vi "6009_short.vi"() -> ()   [LabVIEW 2009]
panel:
  out "Waveform Graph 2":dynamicdata(graph)
  out "Waveform Graph":dynamicdata(graph)
  in  "stop (F)":bool
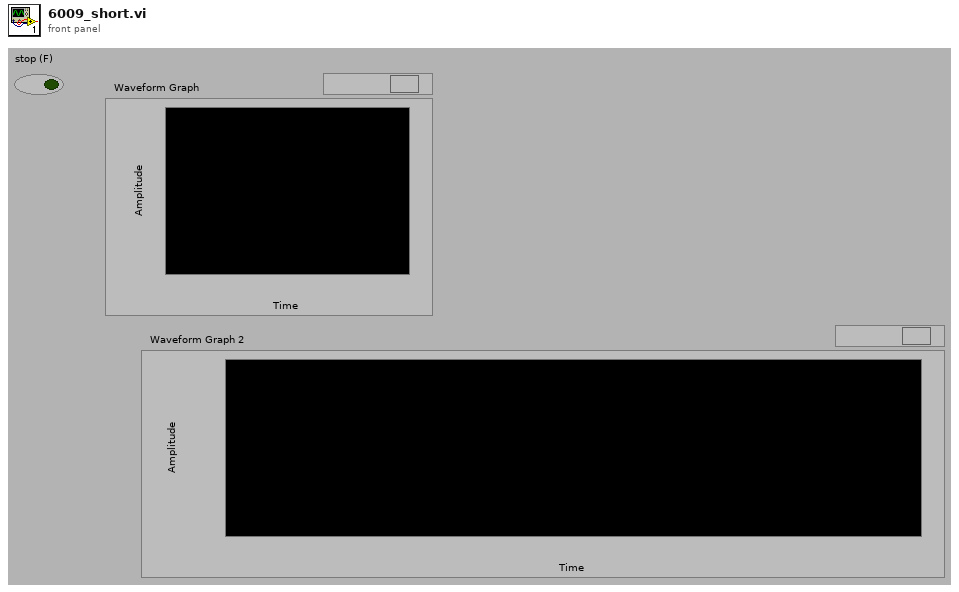
[diagram p1: front panel]
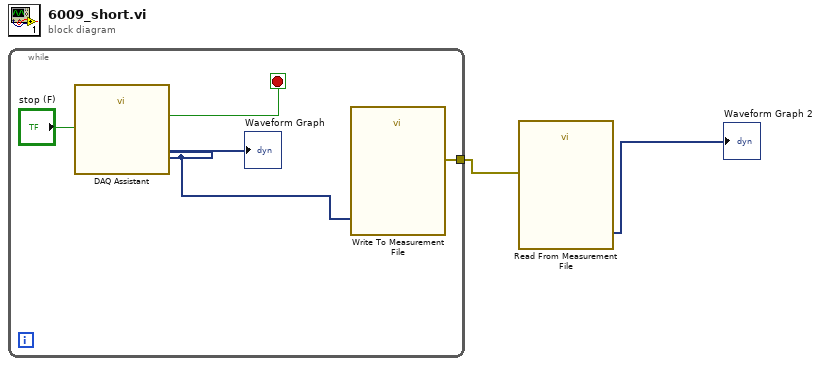
[diagram p0: block diagram]
diagram:
  n1 = while {
    tunnel: [w3] -> w2
    stop <- w5 stop-if-true
    n2 = call "DAQ Assistant"("stop (F)"="stop (F)") -> ("data"=w4:dynamicdata, "stopped"=w5:bool)  [unwired: 15 in, 2 out]
    "Waveform Graph" <- w4
    n3 = call "Write To Measurement File"("Signals"=w4) -> ("error out"=w3:errorcluster)  [unwired: 16 in, 2 out]
  }
  n4 = call "Read From Measurement File"("error in (no error)"=w2) -> ("Signals"=→"Waveform Graph 2":dynamicdata)  [unwired: 5 in, 5 out]
